vi "Демультиплексор.vi"(6 "C / WR":bool, 7 "adrA":cluster{"h1":bool, "h0":bool}) -> (3 "Cluster":T1)   [LabVIEW 2017]
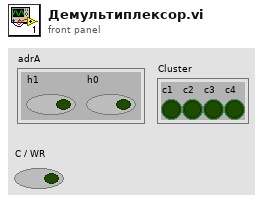
[diagram p1: front panel]
types:
  T1 = cluster{"c1":bool, "c2":bool, "c3":bool, "c4":bool}
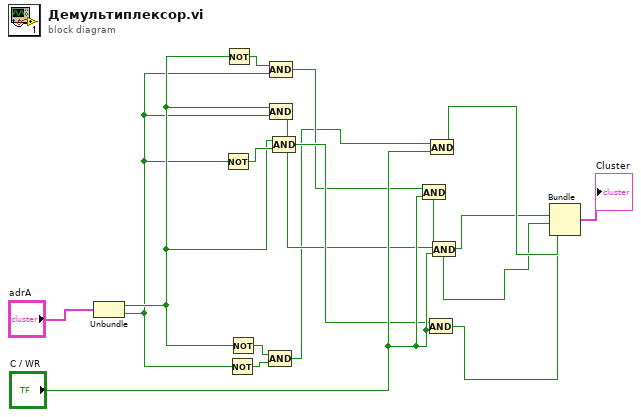
[diagram p0: block diagram]
diagram:
  n1 = Unbundle("adrA") -> ("h1"=w13:bool, "h0"=w12:bool)
  n2 = Not(x=w12) -> (.not. x?=w16:bool)
  n3 = Not(x=w13) -> (.not. x?=w15:bool)
  n4 = Not(x=w12) -> (.not. x?=w11:bool)
  n5 = Not(x=w13) -> (.not. x?=w14:bool)
  n6 = Compound Arithmetic op=AND(w14, w11) -> (w6:bool)
  n7 = Compound Arithmetic op=AND(w15, w12) -> (w7:bool)
  n8 = Compound Arithmetic op=AND(w13, w12) -> (w8:bool)
  n9 = Compound Arithmetic op=AND(w13, w16) -> (w9:bool)
  n10 = And(x=w7, y="C / WR") -> (x .and. y?=w4:bool)
  n11 = And(x=w9, y="C / WR") -> (x .and. y?=w2:bool)
  n12 = And(x=w6, y="C / WR") -> (x .and. y?=w5:bool)
  n13 = And(x=w8, y="C / WR") -> (x .and. y?=w3:bool)
  n14 = Bundle(w5, w4, w3, w2) -> (→"Cluster":cluster{bool, bool, bool, bool})  [unwired: 1 in]
